vi "Set Ref Clock Source.vi"(8 "error in (no error)":errorcluster, 10 "Reference Source (T: Internal)":bool=TRUE, 11 "VISA resource name":refnum<visa-resource-name>) -> (0 "error out":errorcluster, 3 "VISA resource name out":refnum<visa-resource-name>)   [LabVIEW 2020, in "Fluke 5XXX Series Multicalibrators.lvlib"]
doc: "This VI sets the reference clock source (internal or through the 10 MHz IN BNC connector). Once set, the Calibrator retains the external guard setting until power off or reset.\n\nNote:\n\nThis VI is available only for instrument model 5520A."
uses:
  Fluke 5XXX Series Multicalibrators.lvlib
panel:
  # "Internal"
  # "External"
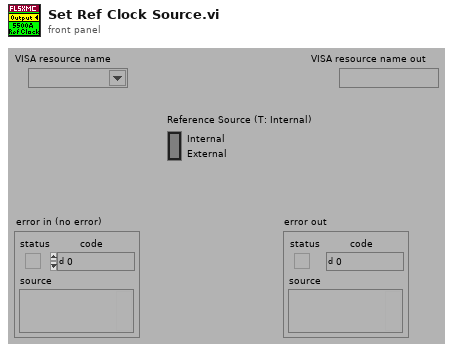
[diagram p1: front panel]
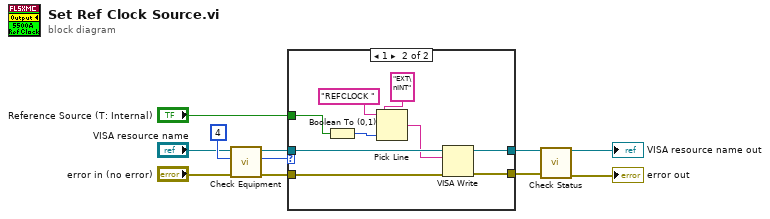
[diagram p0: block diagram]
diagram:
  n1 = call "Check Equipment.vi"("error in (no error)"="error in (no error)", "Bit Mask"=4 ("Numeric"), "VISA resource name"="VISA resource name") -> ("error out"=w9:errorcluster, "Present?"=w8:u32, "VISA resource name out"=w7:refnum<visa-resource-name>)  [unwired: 6 in]
  n2 = case shown="1" w8 {
    tunnel: "Reference Source (T: Internal)" -> [_ w19]
    tunnel: [w12 w17] -> w10
    tunnel: w9 -> [w13 w16]
    tunnel: w7 -> [w12 w15]
    tunnel: [w13 w18] -> w6
    frame 0, Default {
    }
    frame 1 {
      n3 = Boolean To (0,1)(Boolean=w19) -> (0, 1=w20:i16)
      n4 = Pick Line(string ("")="REFCLOCK " ("Reset Command"), multi-line string="EXT\nINT", line index=w20) -> (output string=w14:string)
      n5 = VISA Write(VISA resource name=w15, write buffer=w14, error in (no error)=w16) -> (VISA resource name out=w17:refnum<visa-resource-name>, error out=w18:errorcluster)  [unwired: 1 out]
    }
  }
  n6 = call "Check Status.vi"("VISA resource name"=w10, "error in (no error)"=w6) -> ("VISA resource name out"=→"VISA resource name out":refnum<visa-resource-name>, "error out"=→"error out":errorcluster)  [unwired: 12 in]
